vi "ATS9350_AsyncDMA.vi"() -> ()   [LabVIEW 2012]
doc: "ATS_AutoDMA.vi:\nExample of using the AutoDMA mode."
uses:
  ATS_ctl/ATS_DMA_Channel.ctl
  ATS_ctl/ATS_ReadSamples.ctl
  ATS_ctl/Device_Ctrl.ctl
  ATS_ctl/ATS_Async_Ctrl.ctl
  ATS_ctl/ATS_Check_Ctrl.ctl
  ATS_ctl/ClockSource.ctl
  ATS_ctl/ClockEdge.ctl
  ATS_ctl/Coupling.ctl
  ATS_ctl/Impedance.ctl
  ATS_ctl/TriggerOperation.ctl
  ATS_ctl/Bandwidth.ctl
  ATS_ctl/ExtTrigRange.ctl
  ATS_ctl/ATS_Async_Setting.ctl
  ATS_ctl/ATS_Async_Mode.ctl
panel:
  in  "Case Constant\n(See Context Help)":bool=TRUE
  in  "GetProcessedData":bool=TRUE
  in  "DataBuffer":bool
  out "Board":string
  in  "VersionC":bool caption="Version"
  out "Version":string=" "
  in  "Buffer Count":i32
  in  "StopCapture":bool
  in  "Tab Control":T1(tab)=enum."NPT"
  in  "Trad_ReadSamples":T2={"Offset"=0, "Length"=8192} caption="ReadSamples"
  in  "Trad_Records":u32=100 caption="Total Records"
  in  "Trad_RecPerBuf":u32=1 caption="RecPerBuf"
  out "NPT_BufferSize":u32=1024000 caption="BufferSize"
  in  "NPT_RecLength":u32=8192 caption="Record Length"
  in  "NPT_TotalRecords":u32=10000 caption="Total Records"
  in  "NPT_RecPerBuf":u32=125 caption="Records Per Buffer"
  in  "CT_Records":u32=100 caption="Total Records"
  in  "CT_BufferSize":u32=1024000 caption="Buffer Size"
  in  "TR_Records":u32=100 caption="Total Records"
  in  "Trig_BufferSize":u32=1024000 caption="Buffer Size"
  in  "SetupDMA":bool
  out "Error":string
  out "cFlags":u32 format="%x"
  out "SR (S/s)":dbl=10000000.0 format="%.2p"
  out "#Records":i32
  out "#Valid Buffer":i32
  out "ready":bool
  in  "SetBoard":bool
  in  "StartCapture":bool
  in  "Display":bool
  in  "Write TO file":bool
  out "#Loop":i32
  out "Time (ms)":u32
  out "Waveform Graph":u16[][](graph)
  out "Return Code":u32
  out "ReadSamples_Out":T2
  in  "Channel":T3
  in  "Device":i32
  in  "Stop":bool
  # "Total_Rec = 0 ==> Infini"
  # "Warning: Do not use ATS9462 in Traditional Mode"
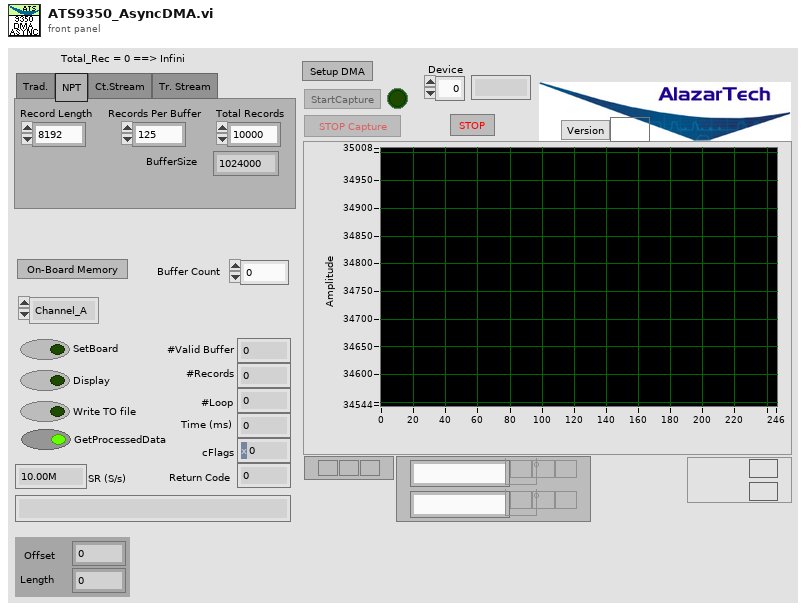
[diagram p1: front panel]
types:
  T1 = enum32{"Trad.", "NPT", "Ct.Stream", "Tr. Stream"}
  T2 = typedef "ATS_ReadSamples.ctl" = cluster{"Offset":i32, "Length":u32}
  T3 = typedef "ATS_DMA_Channel.ctl" = enum16{"Channel_A", "Channel_B", "A & B"}
  T4 = typedef "Device_Ctrl.ctl" = enum16{"Status", "About", "Arm", "ForceTrig", "Abort", "Initialize", "Init (NoPreset)", "Info", "Close", "Calibrate", "SetManually", "LED_ON", "LED_OFF"}
  T5 = typedef "ATS_Async_Ctrl.ctl" = enum16{"SetupDMA", "StartCapture", "Get", "Get_Stream", "Abort", "Stop"}
  T6 = typedef "ATS_Check_Ctrl.ctl" = enum16{"None", "NO_ATS9462", "ATS9462_Traditional", "Verify Board", "OnBoard Memory", "Board & Memory", "Master/Slave", "NO Master/Slave"}
  T7 = typedef "ATS_Async_Setting.ctl" = cluster{"UseHeader":u32, "Rec/Buffer":u32, "Total_Rec":u32, "DataBuffer":bool, "GetProcessedData":bool}
  T8 = typedef "ATS_Async_Mode.ctl" = enum16{"Continuous", "Triggered", "No-Pre-Trigger", "Traditional"}
  T9 = cluster{"Stop":bool, "Write TO file":bool, "SetBoard":bool, "StartDMA":bool, "StartCapture":bool, "Version":bool}
  T10 = cluster{"Stop":bool, "Write TO file":bool, "SetBoard":bool, "SetupDMA":bool, "StartCapture":bool, "VersionC":bool}
  T11 = cluster{"Stop":bool, "Write TO file":bool, "SetBoard":bool, bool, "StartCapture":bool, bool}
  T12 = typedef "ATS_Global.ctl" = cluster{"Record":T13, "Clock":T14, "Input A":T18, "Input B":T18, "Trigger":T23}
  T13 = typedef "Record.ctl" = cluster{"Count":u32, "Presize":u32, "Length":u32}
  T14 = typedef "Clock.ctl" = cluster{"ClckSource":T15, "ClckRate":T16, "ClckEdge":T17, "Decimation":u32}
  T15 = typedef "ClockSource.ctl" = enum16{"Internal", "External", "Medium Ext.", "Slow Ext.", "Ext. AC", "Ext. DC", "Ext. (PLL)"}
  T16 = typedef "ClockRate.ctl" = u32
  T17 = typedef "ClockEdge.ctl" = u16
  T18 = typedef "InputCtrl.ctl" = cluster{"Coupling":T19, "Range":T20, "Impedance":T21, "Bandwidth":T22}
  T19 = typedef "Coupling.ctl" = enum16{"AC", "DC"}
  T20 = typedef "Range.ctl" = u32
  T21 = typedef "Impedance.ctl" = enum16{"1M ohms", "50 ohms"}
  T22 = typedef "Bandwidth.ctl" = enum16{"Full Bandwidth", "Reduce Bandwidth"}
  T23 = typedef "Trigger.ctl" = cluster{"TrigOperation":T24, "Timeout (s)":dbl, "Trig. Delay":u32, "Engine X":T25, "Engine Y":T25, "ExtTrigControl":T26}
  T24 = typedef "TriggerOperation.ctl" = enum16{"Only X", "Only Y", "X or Y", "X and Y", "X xor Y", "X and not Y", "not X and Y"}
  T25 = typedef "TriggerEngine.ctl" = cluster{"Source":enum32{"Chan_A", "Chan_B", "External", "Disable"}, "Slope":enum32{"Positive", "Negative"}, "Level":u32}
  T26 = typedef "ExtTrigger.ctl" = cluster{"Coupling":T19, "Range":T27}
  T27 = typedef "ExtTrigRange.ctl" = enum16{"1 V", "5 V", "TTL"}
  T28 = cluster{"DeviceOut":i32, "Setup_Out":T12, "SR (S/s)":dbl, "Controls":cluster{"Stop":bool, "Write TO file":bool, "SetBoard":bool, "StartDMA":bool, "StartCapture":bool, "Version":bool}, "Flash":bool, "Record/Buf":u32, "BufCount_Out":i32}
  T29 = typedef "ATS_Async_Status.ctl" = cluster{"Start DMA":bool, "StartCapture":bool, "Valid":bool, "Completed":bool, "InProgress":bool, "Timeout":bool, "Overflow":bool, "Error":bool}
  T30 = typedef "Device_Info.ctl" = cluster{"Handle":u32, "Board":string, "CPLD":string, "MemorySize":u32, "SampleSize":u8, "ID":i32, "High_Memory":bool, "Chan/Board":u8}
  T31 = typedef "ATS_Global_Specs_Ctrl.ctl" = cluster{"ClckSource":cluster{"Internal":bool, "External":bool, "Medium Ext.":bool, "Slow Ext.":bool, "Ext. AC":bool, "Ext. DC":bool, "Ext. (PLL)":bool}, "ClckRate":cluster{"1 kS/s":bool, "2 kS/s":bool, "5 kS/s":bool, "10 kS/s":bool, "20 kS/s":bool, "50 kS/s":bool, "100 kS/s":bool, "200 kS/s":bool, "500 kS/s":bool, "1 MS/s":bool, "2 MS/s":bool, "5 MS/s":bool, "10 MS/s":bool, "20 MS/s":bool, "25 MS/s":bool, "50 MS/s":bool, "100 MS/s":bool, "125 MS/s":bool, "160 MS/s":bool, "180 MS/s":bool, "200 MS/s":bool, "250 MS/s":bool, "500 MS/s":bool, "1 GS/s":bool}, "ClckEdge":cluster{"Rising":bool, "Falling":bool}, "InputCoupling":cluster{"AC":bool, "DC":bool}, "InputRange":cluster{"20mV":bool, "40mV":bool, "50mV":bool, "80mV":bool, "100mV":bool, "200mV":bool, "400mV":bool, "500mV":bool, "800mV":bool, "1 V":bool, "2 V":bool, "4 V":bool, "5 V":bool, "8 V":bool, "10 V":bool, "16 V":bool, "20 V":bool, "40 V":bool, "HiFi":bool, "1.25 V":bool}, "Impedance":cluster{"1M ohms":bool, "50 ohms":bool, "300 ohms":bool}, "Bandwidth":cluster{"Full":bool, "Reduce":bool}, "RangeLim(50)":string, "AsyncDMA":cluster{"OnBoard":bool, "FPGA":bool}, "Memory":cluster{"VerifMem":bool, "HighMem":bool, "Combine":bool, "HighRecord":bool}, "ExtTrigCoupling":cluster{"AC":bool, "DC":bool}, "ExtTrigRange":cluster{"1 V":bool, "5 V":bool, "\nTTL":bool}, "AUX_IO_Trig":cluster{"Trig_Out":bool, "Trig_In":bool}, "AUX_IO_Slope":cluster{"Rising":bool, "Falling":bool}, "MaxPretrig":cluster{"MEM":u32, "FIFO":u32}, "AUX_I/O_Trig":cluster{"OUT_Trigger":bool, "OUT_PACER":bool, "OUT_BUSY":bool, "OUT_CLOCK":bool, "OUT_RESERVED":bool, "OUT_CAPTURE_ALMOST_DONE":bool, "OUT_AUXILIARY":bool, "OUT_SERIAL_DATA":bool, "IN_TRIGGER_ENABLE":bool, "IN_DIGITAL_TRIGGER":bool, "IN_GATE":bool, "IN_CAPTURE_ON_DEMAND":bool, "IN_RESET_TIMESTAMP":bool, "IN_SLOW_EXTERNAL_CLOCK":bool, "INPUT_AUXILIARY":bool, "INPUT_SERIAL_DATA":bool}, "ChannelsPerBoard":u8}
  T32 = enum32{"Chan_A", "Chan_B", "External", "Disable"}
  T33 = cluster{"Coupling":T19, "9350_Range":u32, "Impedance":T21, "Bandwidth":T22}
  T34 = cluster{"ClckSource":T15, "9350_ClckRate":u32, "ClckEdge":T17, "Decimation":u32}
  T35 = cluster{"Source":enum32{"Chan_A", "Chan_B", "External", "Disable"}, "Slope":enum32{"Positive", "Negative"}, "Level":u32}
  T36 = cluster{"Engine Relationship":T24, "Timeout (s)":dbl, "Trig. Delay":u32, cluster{"Source":enum32{"Chan_A", "Chan_B", "External", "Disable"}, "Slope":enum32{"Positive", "Negative"}, "Level":u32}, cluster{"Source":enum32{"Chan_A", "Chan_B", "External", "Disable"}, "Slope":enum32{"Positive", "Negative"}, "Level":u32}, cluster{"Coupling":T19, "Range":T27}}
  T37 = cluster{cluster{"Count":u32, "Offset":i32, "Length":u32}, cluster{"ClckSource":T15, "9350_ClckRate":u32, "ClckEdge":T17, "Decimation":u32}, cluster{"Coupling":T19, "9350_Range":u32, "Impedance":T21, "Bandwidth":T22}, cluster{"Coupling":T19, "9350_Range":u32, "Impedance":T21, "Bandwidth":T22}, cluster{"Engine Relationship":T24, "Timeout (s)":dbl, "Trig. Delay":u32, cluster{"Source":enum32{"Chan_A", "Chan_B", "External", "Disable"}, "Slope":enum32{"Positive", "Negative"}, "Level":u32}, cluster{"Source":enum32{"Chan_A", "Chan_B", "External", "Disable"}, "Slope":enum32{"Positive", "Negative"}, "Level":u32}, cluster{"Coupling":T19, "Range":T27}}}
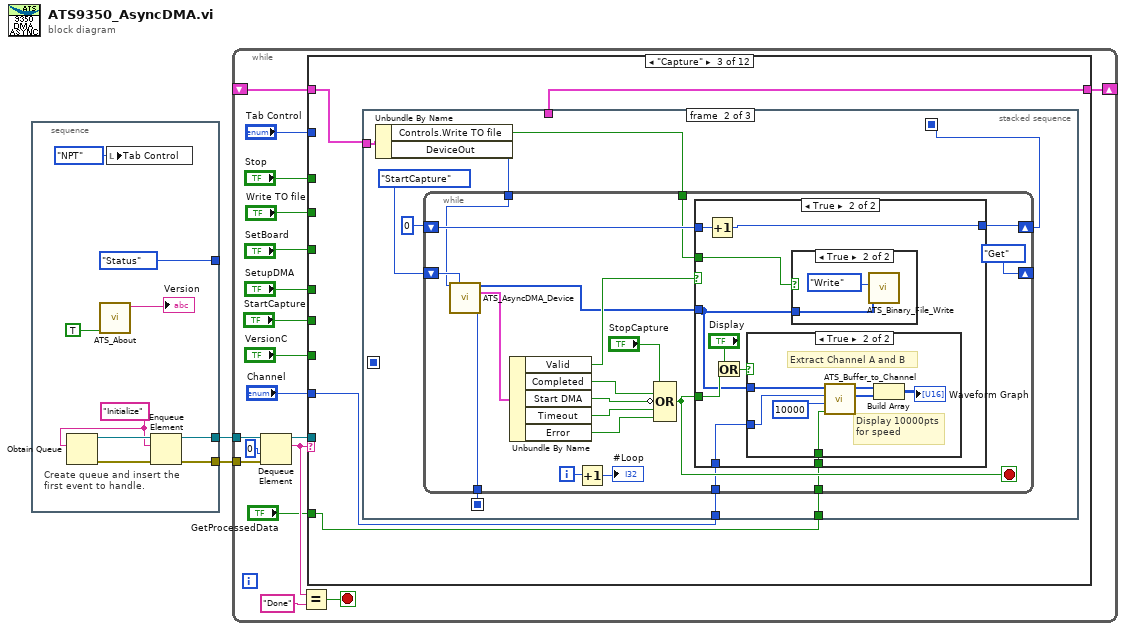
[diagram p0: block diagram]
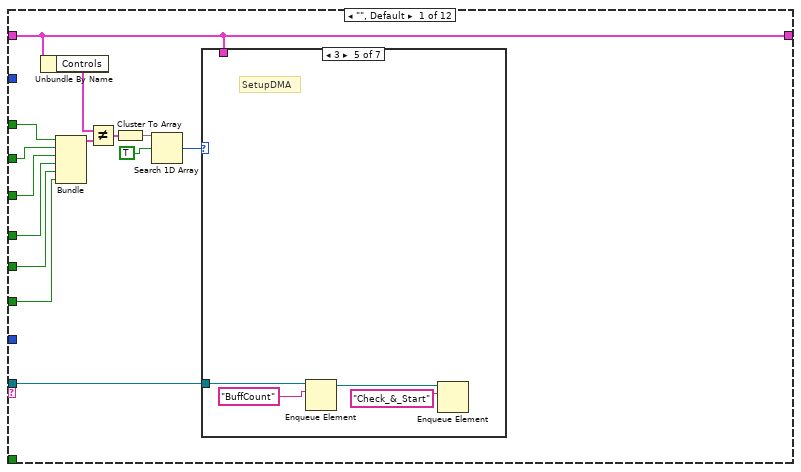
[diagram p2: hidden frame]
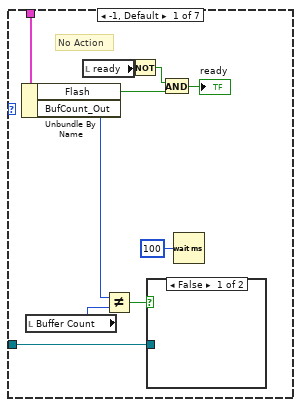
[diagram p3: hidden frame]
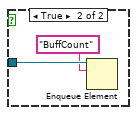
[diagram p4: hidden frame]
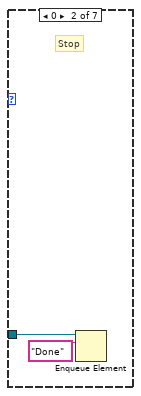
[diagram p5: hidden frame]
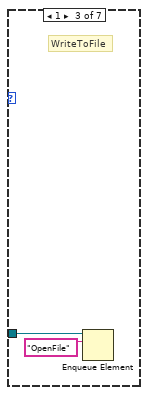
[diagram p6: hidden frame]
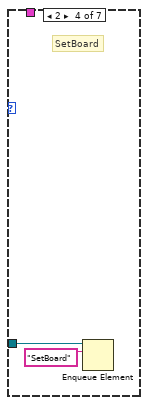
[diagram p7: hidden frame]
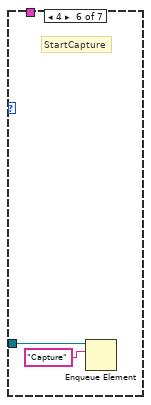
[diagram p8: hidden frame]
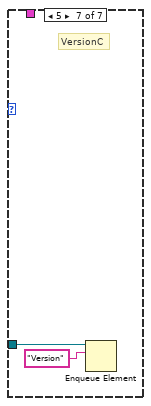
[diagram p9: hidden frame]
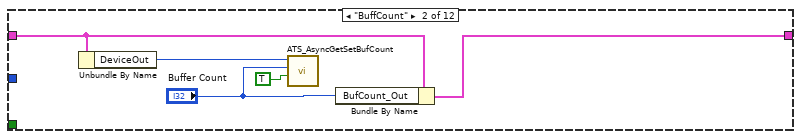
[diagram p10: hidden frame]
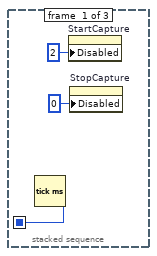
[diagram p11: hidden frame]
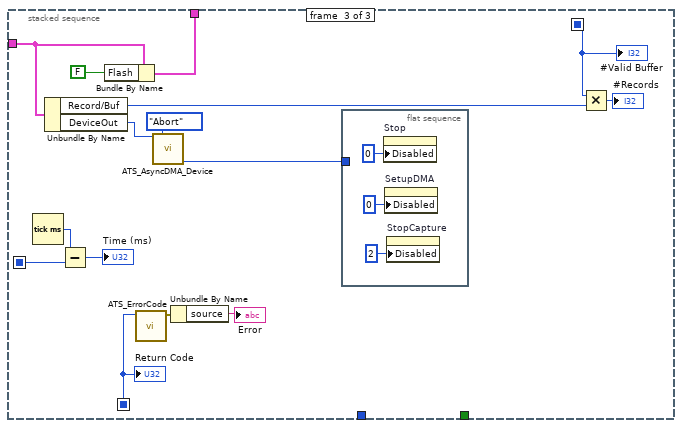
[diagram p15: hidden frame]
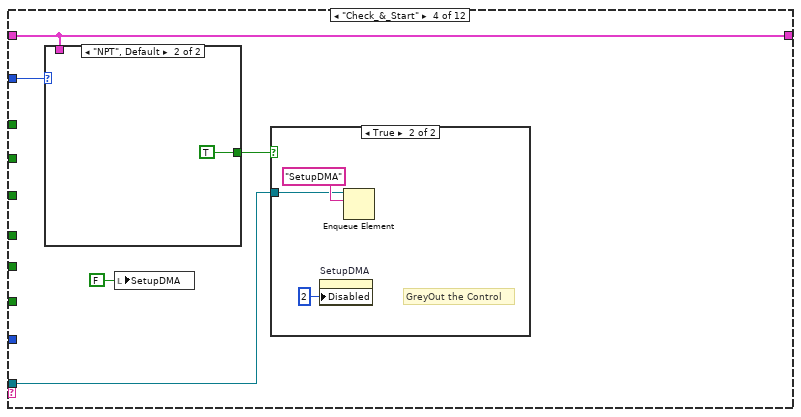
[diagram p16: hidden frame]
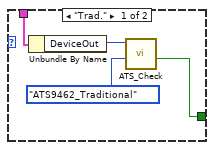
[diagram p18: hidden frame]
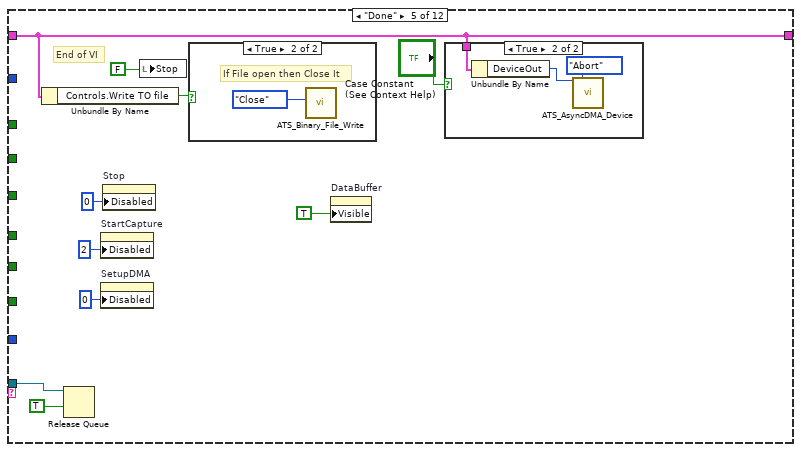
[diagram p19: hidden frame]
diagram:
  n1 = stacked-sequence {
    tunnel: [Device_Ctrl."Status" ("DevCtrl")] -> _
    tunnel: [w8] -> w2
    tunnel: [w7] -> w1
    frame #0 {
      w5 = "Initialize"
      # "Create queue and insert the\nfirst event to handle."
      n2 = Obtain Queue(element data type=w5) -> (queue out=w6:refnum<queue>, error out=w9:errorcluster)  [unwired: 4 in, 1 out]
      n3 = call "ATS_About.vi"("NO Display"=TRUE) -> ("Version#"=→"Version":string)  [unwired: 5 in, 1 out]
      n4 = local write "Tab Control"(T1."NPT" ("Tab Control")) -> ()
      n5 = Enqueue Element(queue=w6, element=w5, error in (no error)=w9) -> (queue out=w8:refnum<queue>, error out=w7:errorcluster)  [unwired: 1 in, 1 out]
    }
  }
  n6 = while {
    tunnel: w2 -> [w27]
    tunnel: w1 -> [w28]
    shift-right: [w22] -> _
    shift-left: _ -> [w21]
    stop <- w26 stop-if-true
    n7 = Dequeue Element(queue=w27, timeout in ms (-1)=0 ("ms timeout (-1)"), error in (no error)=w28) -> (queue out=w23:refnum<queue>, element=w24:string)  [unwired: 2 out]
    n8 = Equal?(x=w24, y="Done") -> (x = y?=w26:bool)
    n9 = case shown="\"Capture\"" w24 {
      tunnel: w23 -> [w35 _ _ w150 w170 w207 _ w254 w262 _ w344 _]
      tunnel: [w31 w73 w77 w152 w167 w204 w217 w257 w266 w292 w348 w350] -> w22
      tunnel: w21 -> [w31 w74 w78 w152 w167 _ w218 w253 w261 w293 w348 w350]
      tunnel: "Write TO file" -> [w43 _ _ _ _ _ w216 _ _ _ _ _]
      tunnel: "SetBoard" -> [w42 _ _ _ _ _ _ _ _ _ _ _]
      tunnel: "SetupDMA" -> [w34 _ _ _ _ _ _ _ _ _ _ _]
      tunnel: "Stop" -> [w33 _ _ _ _ _ _ _ _ _ _ _]
      tunnel: "StartCapture" -> [w32 _ _ _ _ _ _ _ _ _ _ _]
      tunnel: "Channel" -> [_ _ w76 _ _ _ _ _ _ w289 _ _]
      tunnel: "Tab Control" -> [_ _ _ w151 _ _ _ _ _ w271 _ _]
      tunnel: "VersionC" -> [w30 _ _ _ _ _ _ _ _ _ _ _]
      tunnel: "GetProcessedData" -> [_ _ w75 _ _ _ _ _ _ w270 _ _]
      frame "", Default {
        n10 = Unbundle By Name(w31) -> ("Controls"=w40:T9)
        n11 = Bundle("Stop"=w33, "Write TO file"=w43, "SetBoard"=w42, "SetupDMA"=w34, "StartCapture"=w32, "VersionC"=w30) -> (w41:T10)  [unwired: 1 in]
        n12 = Not Equal?(x=w40, y=w41) -> (x != y?=w39:T11)
        n13 = Cluster To Array(cluster=w39) -> (array=w37:bool[])
        n14 = Search 1D Array(1D array=w37, element=TRUE) -> (index of element=w36:i32)  [unwired: 1 in]
        n15 = case shown="3" w36 {
          tunnel: w35 -> [w44 w57 w58 w60 w65 w66 w68]
          tunnel: w31 -> [w52 _ _ _ _ _ _]
          frame -1, Default {
            # "No Action"
            n16 = Unbundle By Name(w52) -> ("Flash"=w49:bool, "BufCount_Out"=w47:i32)
            n17 = local read "Buffer Count"() -> (w46:i32)
            n18 = local read "ready"() -> (w51:bool)
            n19 = Not Equal?(x=w47, y=w46) -> (x != y?=w45:bool)
            n20 = Not(x=w51) -> (.not. x?=w48:bool)
            n21 = case shown="False" w45 {
              tunnel: w44 -> [_ w55]
              frame False {
              }
              frame True {
                n22 = Enqueue Element(queue=w55, element="BuffCount") -> ()  [unwired: 2 in, 3 out]
              }
            }
            n23 = And(x=w48, y=w49) -> (x .and. y?=→"ready":bool)
            n24 = Wait (ms)(milliseconds to wait=u32 100) -> ()  [unwired: 1 out]
          }
          frame 0 {
            # "Stop"
            n25 = Enqueue Element(queue=w57, element="Done") -> ()  [unwired: 2 in, 3 out]
          }
          frame 1 {
            # "WriteToFile"
            n26 = Enqueue Element(queue=w58, element="OpenFile") -> ()  [unwired: 2 in, 3 out]
          }
          frame 2 {
            # "SetBoard"
            n27 = Enqueue Element(queue=w60, element="SetBoard") -> ()  [unwired: 2 in, 3 out]
          }
          frame 3 {
            # "SetupDMA"
            n28 = Enqueue Element(queue=w65, element="BuffCount") -> (queue out=w62:refnum<queue>)  [unwired: 2 in, 2 out]
            n29 = Enqueue Element(queue=w62, element="Check_&_Start") -> ()  [unwired: 2 in, 3 out]
          }
          frame 4 {
            # "StartCapture"
            n30 = Enqueue Element(queue=w66, element="Capture") -> ()  [unwired: 2 in, 3 out]
          }
          frame 5 {
            # "VersionC"
            n31 = Enqueue Element(queue=w68, element="Version") -> ()  [unwired: 2 in, 3 out]
          }
        }
      }
      frame "BuffCount" {
        n32 = Unbundle By Name(w74) -> ("DeviceOut"=w72:i32)
        n33 = call "ATS_AsyncGetSetBufCount.vi"("Get / Set&Get"=TRUE, "BuffCount"="Buffer Count", "DeviceIn"=w72) -> ()  [unwired: 6 in, 3 out]
        n34 = Bundle By Name(cluster=w74, "BufCount_Out"="Buffer Count") -> (w73:T28)
      }
      frame "Capture" {
        n35 = stacked-sequence {
          seq-local: [w81 _ _] -> [_ _ w142]
          seq-local: [_ w85 _] -> [_ _ w132]
          seq-local: [_ w83 _] -> [_ _ w131]
          tunnel: w78 -> [_ w88 w137]
          tunnel: [_ _ w140] -> w77
          tunnel: w76 -> [_ w84 _]
          tunnel: w75 -> [_ w82 _]
          frame #0 {
            n36 = Tick Count (ms)() -> (millisecond timer value=w81:u32)
            n37 = property on="StartCapture" class="Bool"("Disabled"=u8 2) -> ()  [unwired: 2 in, 2 out]
            n38 = property on="StopCapture" class="Bool"("Disabled"=u8 0) -> ()  [unwired: 2 in, 2 out]
          }
          frame #1 {
            n39 = Unbundle By Name(w88) -> ("Controls.Write TO file"=w86:bool, "DeviceOut"=w87:i32)
            n40 = while {
              shift-right: [w101] -> w83
              shift-left: 0 -> [w105]
              shift-right: [ATS_Async_Ctrl."Get" ("ATS_DMA_Ctrl")] -> _
              shift-left: ATS_Async_Ctrl."StartCapture" ("ATS_DMA_Ctrl") -> [w99]
              tunnel: [w97] -> w85
              tunnel: w87 -> [w96]
              tunnel: w86 -> [w95]
              tunnel: w84 -> [w94]
              tunnel: w82 -> [w91]
              i -> [w106]
              stop <- w103 stop-if-true
              n41 = call "ATS_AsyncDMA_Device.vi"("DeviceIn"=w96, "ATS_Async_Ctrl"=w99) -> ("Buffer"=w107:u16[], "Async_Status"=w92:T29, "Return Code"=w97:u32)  [unwired: 9 in, 2 out]
              n42 = Unbundle By Name(w92) -> ("Valid"=w110:bool, "Completed"=w104:bool, "Start DMA"=w109:bool, "Timeout"=w108:bool, "Error"=w98:bool)
              n43 = Increment(x=w106) -> (x+1=→"#Loop":i32)
              n44 = Compound Arithmetic op=OR("StopCapture", w104, invert w109, w108, w98) -> (w103:bool)
              n45 = case shown="True" w110 {
                tunnel: w107 -> [_ w115]
                tunnel: w95 -> [_ w120]
                tunnel: w105 -> [w111 w118]
                tunnel: [w111 w114] -> w101
                tunnel: w103 -> [_ w116]
                tunnel: w94 -> [_ w113]
                tunnel: w91 -> [_ w112]
                frame False {
                }
                frame True {
                  n46 = Increment(x=w118) -> (x+1=w114:i32)
                  n47 = Or(x="Display", y=w116) -> (x .or. y?=w117:bool)
                  n48 = case shown="True" w117 {
                    tunnel: w115 -> [_ w123]
                    tunnel: w113 -> [_ w122]
                    tunnel: w112 -> [_ w121]
                    frame False {
                    }
                    frame True {
                      # "Extract Channel A and B"
                      # "Display 10000pts\nfor speed"
                      n49 = call "ATS_Buffer_to_Channel.vi"("GetProcessedData"=w121, "MaxLength (-1)"=10000 ("length"), "Channel"=w122, "Buffer [AB]"=w123) -> ("[B]"=w126:u16[], "[A]"=w127:u16[])  [unwired: 6 in]
                      n50 = Build Array(w127, w126) -> (→"Waveform Graph":u16[][])
                    }
                  }
                  n51 = case shown="True" w120 {
                    tunnel: w115 -> [_ w128]
                    frame False {
                    }
                    frame True {
                      n52 = call "ATS_Binary_File_Write.vi"("Data_In"=w128, "Write_Ctrl"=enum16{"Open", "Write", "Close"}."Write") -> ()  [unwired: 8 in, 2 out]
                    }
                  }
                }
              }
            }
          }
          frame #2 {
            n53 = Tick Count (ms)() -> (millisecond timer value=w144:u32)
            n54 = Unbundle By Name(w137) -> ("Record/Buf"=w135:u32, "DeviceOut"=w134:i32)
            n55 = Subtract(x=w144, y=w142) -> (x-y=→"Time (ms)":u32)
            n56 = Bundle By Name(cluster=w137, "Flash"=FALSE) -> (w140:T28)
            n57 = call "ATS_ErrorCode.vi"("ErrorCode"=w132) -> ("error out"=w133:errorcluster)  [unwired: 6 in]
            n58 = call "ATS_AsyncDMA_Device.vi"("DeviceIn"=w134, "ATS_Async_Ctrl"=ATS_Async_Ctrl."Abort" ("ATS_DMA_Ctrl")) -> ("Return Code"=w130:u32)  [unwired: 9 in, 4 out]
            n59 = Unbundle By Name(w133) -> ("source"=→"Error":string)
            n60 = flat-sequence {
              tunnel: w130 -> [_]
              frame #0 {
                n61 = property on="Stop" class="Bool (strict)"("Disabled"=u8 0) -> ()  [unwired: 2 in, 2 out]
                n62 = property on="SetupDMA" class="Bool (strict)"("Disabled"=u8 0) -> ()  [unwired: 2 in, 2 out]
                n63 = property on="StopCapture" class="Bool"("Disabled"=u8 2) -> ()  [unwired: 2 in, 2 out]
              }
            }
            n64 = Multiply(x=w131, y=w135) -> (x*y=→"#Records":u32)
            "Return Code" <- w132
            "#Valid Buffer" <- w131
          }
        }
      }
      frame "Check_&_Start" {
        n65 = case shown="\"NPT\", Default" w151 {
          tunnel: w152 -> [w159 _]
          tunnel: [w157 TRUE ("OK")] -> w149
          frame "Trad." {
            n66 = Unbundle By Name(w159) -> ("DeviceOut"=w158:i32)
            n67 = call "ATS_Check.vi"("ATS_Check"=ATS_Check_Ctrl."ATS9462_Traditional", "Device"=w158) -> ("OK"=w157:bool)  [unwired: 8 in, 1 out]
          }
          frame "NPT", Default {
          }
        }
        n68 = local write "SetupDMA"(FALSE ("StartDMA")) -> ()
        n69 = case shown="True" w149 {
          tunnel: w150 -> [_ w154]
          frame False {
          }
          frame True {
            # "GreyOut the Control"
            n70 = property on="SetupDMA" class="Bool (strict)"("Disabled"=u8 2) -> ()  [unwired: 2 in, 2 out]
            n71 = Enqueue Element(queue=w154, element="SetupDMA") -> ()  [unwired: 2 in, 3 out]
          }
        }
      }
      frame "Done" {
        # "End of VI"
        n72 = Unbundle By Name(w167) -> ("Controls.Write TO file"=w168:bool)
        n73 = Release Queue(queue=w170, force destroy? (F)=TRUE) -> ()  [unwired: 1 in, 3 out]
        n74 = property on="StartCapture" class="Bool"("Disabled"=u8 2) -> ()  [unwired: 2 in, 2 out]
        n75 = property on="SetupDMA" class="Bool (strict)"("Disabled"=u8 0) -> ()  [unwired: 2 in, 2 out]
        n76 = property on="Stop" class="Bool (strict)"("Disabled"=u8 0) -> ()  [unwired: 2 in, 2 out]
        n77 = local write "Stop"(FALSE ("Stop")) -> ()
        n78 = case shown="True" w168 {
          frame False {
          }
          frame True {
            # "If File open then Close It"
            n79 = call "ATS_Binary_File_Write.vi"("Write_Ctrl"=enum16{"Open", "Write", "Close"}."Close" ("f")) -> ()  [unwired: 9 in, 2 out]
          }
        }
        n80 = property on="DataBuffer" class="Bool (strict)"("Visible"=TRUE) -> ()  [unwired: 2 in, 2 out]
        n81 = case shown="True" "Case Constant\n(See Context Help)" {
          tunnel: w167 -> [_ w172]
          frame False {
          }
          frame True {
            n82 = Unbundle By Name(w172) -> ("DeviceOut"=w171:i32)
            n83 = call "ATS_AsyncDMA_Device.vi"("DeviceIn"=w171, "ATS_Async_Ctrl"=ATS_Async_Ctrl."Abort" ("ATS_DMA_Ctrl")) -> ()  [unwired: 9 in, 5 out]
          }
        }
      }
      frame "Initialize" {
        w190 = u32 0  # Record/Buf
        w203 = T9 {"Stop"=FALSE, "Write TO file"=FALSE, "SetBoard"=FALSE, "StartDMA"=FALSE, "StartCapture"=FALSE, "Version"=FALSE}  # Controls
        w192 = FALSE  # Flash
        # "Reset all Boards"
        n84 = Enqueue Element(queue=w207, element="PreSet" ("queue element")) -> ()  [unwired: 2 in, 3 out]
        n85 = call "ATS_Device.vi"("BoardToVerify"="ATS9350", "ATS_Check"=ATS_Check_Ctrl."Verify Board", "DevCtrl"=Device_Ctrl."Initialize", "DeviceIn"="Device") -> ("DeviceOut"=w209:i32, "DevInfo"=w186:T30)  [unwired: 1 in, 5 out]
        n86 = local write "#Valid Buffer"(0 ("#Valid Buffer")) -> ()
        n87 = local write "#Records"(0 ("#Records")) -> ()
        n88 = Unbundle By Name(w186) -> ("Board"=→"Board":string)
        n89 = property on="StartCapture" class="Bool"("Disabled"=u8 2) -> ()  [unwired: 2 in, 2 out]
        n90 = property on="StopCapture" class="Bool"("Disabled"=u8 2) -> ()  [unwired: 2 in, 2 out]
        n91 = property on="SetupDMA" class="Bool (strict)"("Disabled"=u8 0) -> ()  [unwired: 2 in, 2 out]
        n92 = local write "Time (ms)"(u32 0 ("TimeLoop (ms)")) -> ()
        n93 = property on="Stop" class="Bool (strict)"("Disabled"=u8 0) -> ()  [unwired: 2 in, 2 out]
        n94 = call "ATS_Device.vi"("DevCtrl"=Device_Ctrl."Abort", "DeviceIn"=w209) -> ("DeviceOut"=w181:i32)  [unwired: 3 in, 6 out]
        n95 = call "ATS_Specs_Selection.vi"("Device"=w181) -> ("Specifications"=w180:T31)  [unwired: 4 in, 6 out]
        n96 = call "ATS_MS_Set_Device.vi"("Update_Only"=TRUE ("Set_Manually (F)"), "DeviceIn"=w181) -> ("Setup_Out"=w194:T12, "DeviceOut"=w188:i32)  [unwired: 4 in, 4 out]
        n97 = Unbundle By Name(w180) -> ("AsyncDMA.OnBoard"=w179:bool, "AsyncDMA.FPGA"=w175:bool)
        n98 = call "ATS_AsyncGetSetBufCount.vi"("DeviceIn"=w188) -> ("BufCount_Out"=w187:i32)  [unwired: 8 in, 2 out]
        n99 = local read "SR (S/s)"() -> (w205:dbl)
        n100 = And(x=w179, y=w175) -> (x .and. y?=w178:bool)
        n101 = Unbundle By Name(w203) -> ("Stop"=w196:bool, "Write TO file"=w202:bool, "SetBoard"=w201:bool, "StartDMA"=w197:bool)
        n102 = case shown="False" w178 {
          selector: w178 -> [w213 w215]
          tunnel: [w213 w215] -> w177
          tunnel: [w212 w214] -> w176
          tunnel: w175 -> [w212 w214]
          frame False {
          }
          frame True {
          }
        }
        n103 = local write "Buffer Count"(w187) -> ()
        n104 = Bundle("DeviceOut"=w181, "Setup_Out"=w194, "SR (S/s)"=w205, "Controls"=w203, "Flash"=w192, "Record/Buf"=w190, "BufCount_Out"=w187) -> (w204:T28)  [unwired: 1 in]
        n105 = local write "SetupDMA"(w197) -> ()
        n106 = local write "Write TO file"(w202) -> ()
        n107 = local write "SetBoard"(w201) -> ()
        n108 = local write "Stop"(w196) -> ()
        n109 = property on="DataBuffer" class="Bool (strict)"("Visible"=w177, "Value"=w176) -> ()  [unwired: 2 in, 2 out]
      }
      frame "OpenFile" {
        n110 = Select(t=enum16{"Open", "Write", "Close"}."Open" ("Write_Ctrl"), s=w216, f=enum16{"Open", "Write", "Close"}."Close") -> (s? t:f=w220:enum16{"Open", "Write", "Close"})
        n111 = Bundle By Name(cluster=w218, "Controls.Write TO file"=w216) -> (w217:T28)
        n112 = call "ATS_Binary_File_Write.vi"("Write_Ctrl"=w220) -> ()  [unwired: 9 in, 2 out]
      }
      frame "PreSet" {
        w243 = enum32{"Positive", "Negative"}."Positive"  # Slope
        w242 = enum32{"Positive", "Negative"}."Positive"  # Slope
        w241 = T32."Disable"  # Source
        w239 = T32."Chan_A"  # Source
        w223 = u32 4 items=["40mV", "100mV", "200mV", "400mV", "1 V", "2 V", "4 V"]  # 9350_Range
        w222 = u32 17 items=["1 kS/s", "2 kS/s", "5 kS/s", "10 kS/s", "20 kS/s", "50 kS/s", "100 kS/s", "200 kS/s", "500 kS/s", "1 MS/s", "2 MS/s", "5 MS/s", "10 MS/s", "20 MS/s", "50 MS/s", "100 MS/s", "250 MS/s", "500 MS/s"]  # 9350_ClckRate
        w248 = ExtTrigRange."1 V"  # Range
        w247 = Coupling."AC"  # Coupling
        w246 = Bandwidth."Full Bandwidth"  # Bandwidth
        w245 = u32 0  # Decimation
        w244 = u32 1  # Count
        w227 = u32 0  # Trig. Delay
        w228 = TriggerOperation."Only X"  # Engine Relationship
        w226 = 0.0  # Timeout (s)
        w240 = u32 150  # Level
        w234 = Impedance."50 ohms"  # Impedance
        w232 = Coupling."DC"  # Coupling
        w231 = T17 0 items=["Rising", "Falling"]  # ClckEdge
        w230 = ClockSource."Internal"  # ClckSource
        n113 = Unbundle By Name(w253) -> ("DeviceOut"=w256:i32)
        n114 = Enqueue Element(queue=w254, element="Update" ("queue element")) -> ()  [unwired: 2 in, 3 out]
        n115 = local read "Trad_ReadSamples"() -> (w224:T2)
        n116 = Bundle("Coupling"=w232, "9350_Range"=w223, "Impedance"=w234, "Bandwidth"=w246) -> (w233:T33)  [unwired: 1 in]
        n117 = Bundle("ClckSource"=w230, "9350_ClckRate"=w222, "ClckEdge"=w231, "Decimation"=w245) -> (w235:T34)  [unwired: 1 in]
        n118 = Unbundle By Name(w224) -> ("Offset"=w251:i32, "Length"=w250:u32)
        n119 = Bundle "EngineX"("Source"=w239, "Slope"=w243, "Level"=w240) -> (w237:T35)  [unwired: 1 in]
        n120 = Bundle "EngineY"("Source"=w241, "Slope"=w242, "Level"=w240) -> (w238:T35)  [unwired: 1 in]
        n121 = Bundle("Count"=w244, "Offset"=w251, "Length"=w250) -> (w229:cluster{"Count":u32, "Offset":i32, "Length":u32})  [unwired: 1 in]
        n122 = Bundle "Ext Trig"("Coupling"=w247, "Range"=w248) -> (w249:cluster{"Coupling":T19, "Range":T27})  [unwired: 1 in]
        n123 = Bundle("Engine Relationship"=w228, "Timeout (s)"=w226, "Trig. Delay"=w227, w237, w238, w249) -> (w236:T36)  [unwired: 1 in]
        n124 = Bundle(w229, w235, w233, w233, w236) -> (w225:T37)  [unwired: 1 in]
        n125 = call "ATS_MS_Set_Device.vi"("Set_Manually (F)"=FALSE, "Setup_In"=w225, "DeviceIn"=w256) -> ("Clock_Value (s)"=w252:dbl, "Setup_Out"=w258:T12)  [unwired: 3 in, 4 out]
        n126 = Bundle By Name(cluster=w253, "Setup_Out"=w258, "SR (S/s)"=w252) -> (w257:T28)
      }
      frame "SetBoard" {
        n127 = Unbundle By Name(w261) -> ("DeviceOut"=w264:i32)
        n128 = Enqueue Element(queue=w262, element="Update" ("queue element")) -> ()  [unwired: 2 in, 3 out]
        n129 = local write "SetBoard"(FALSE ("SetBoard")) -> ()
        n130 = call "ATS_MS_Set_Device.vi"("Set_Manually (F)"=TRUE, "DeviceIn"=w264) -> ("Clock_Value (s)"=w265:dbl, "Setup_Out"=w267:T12)  [unwired: 4 in, 4 out]
        n131 = Bundle By Name(cluster=w261, "Setup_Out"=w267, "SR (S/s)"=w265) -> (w266:T28)
      }
      frame "SetupDMA" {
        n132 = case shown="\"NPT\", Default" w271 {
          tunnel: [w302 "Trad_RecPerBuf" u32 1 u32 1] -> w280
          tunnel: ["NPT_TotalRecords" "Trad_Records" "CT_Records" "TR_Records"] -> w281
          tunnel: [ATS_Async_Mode."No-Pre-Trigger" ("Async_Mode") ATS_Async_Mode."Traditional" ("Async_Mode") ATS_Async_Mode."Continuous" ("Async_Mode") ATS_Async_Mode."Triggered" ("Async_Mode")] -> w284
          tunnel: [u32 0 u32 0 u32 0 u32 0] -> w282
          tunnel: [0 ("Offset") w316 0 ("Offset") 0 ("Offset")] -> w287
          tunnel: ["NPT_RecLength" w315 "CT_BufferSize" "Trig_BufferSize"] -> w286
          tunnel: [TRUE ("Start Now / Wait") TRUE ("Start Now / Wait") TRUE ("Start Now / Wait") TRUE ("Start Now / Wait")] -> w269
          frame "NPT", Default {
            n133 = case shown="1, Default" "NPT_TotalRecords" {
              tunnel: "NPT_RecPerBuf" -> [w308 w311]
              tunnel: "NPT_TotalRecords" -> [_ w310]
              tunnel: [w308 w309] -> w302
              frame 0 {
              }
              frame 1, Default {
                n134 = Max & Min(x=w311, y=w310) -> (min(x,y)=w309:u32)  [unwired: 1 out]
                n135 = local write "NPT_RecPerBuf"(w309) -> ()
              }
            }
            n136 = Multiply(x=w302, y="NPT_RecLength") -> (x*y=→"NPT_BufferSize":u32)
          }
          frame "Trad." {
            n137 = Unbundle By Name("Trad_ReadSamples") -> ("Offset"=w316:i32, "Length"=w315:u32)
          }
          frame "Ct.Stream" {
          }
          frame "Tr. Stream" {
          }
        }
        n138 = local write "SetupDMA"(FALSE ("StartDMA")) -> ()
        n139 = Unbundle By Name(w293) -> ("DeviceOut"=w274:i32)
        n140 = Bundle By Name(cluster=T7 {"UseHeader"=0, "Rec/Buffer"=0, "Total_Rec"=0, "DataBuffer"=FALSE, "GetProcessedData"=FALSE} ("Async_Setting"), "UseHeader"=w282, "Rec/Buffer"=w280, "Total_Rec"=w281, "DataBuffer"="DataBuffer", "GetProcessedData"=w270) -> (w279:T7)
        n141 = Bundle By Name(cluster=T2 {"Offset"=0, "Length"=8192} ("Trad_ReadSamples"), "Offset"=w287, "Length"=w286) -> (w285:T2)
        n142 = call "ATS_AsyncDMA_Device.vi"("DeviceIn"=w274, "ATS_Async_Ctrl"=ATS_Async_Ctrl."SetupDMA" ("ATS_DMA_Ctrl"), "Async_Mode"=w284, "Async_Setting"=w279, "Channel"=w289, "ReadSamples"=w285, "Start Now / Wait"=w269) -> ("Async_Status"=w296:T29, "ReadSamples_Out"=w272:T2, "cFlags_Out"=→"cFlags":u32, "Return Code"=w276:u32)  [unwired: 4 in, 1 out]
        "ReadSamples_Out" <- w272
        n143 = case shown="\"Trad.\"" w271 {
          tunnel: w272 -> [w298 _]
          frame "Trad." {
            n144 = local write "Trad_ReadSamples"(w298) -> ()
          }
          frame "NPT", Default {
          }
        }
        n145 = call "ATS_ErrorCode.vi"("ErrorCode"=w276) -> ("error out"=w277:errorcluster)  [unwired: 6 in]
        n146 = local write "Return Code"(w276) -> ()
        n147 = Unbundle By Name(w277) -> ("source"=w278:string)
        n148 = Unbundle By Name(w296) -> ("Error"=w291:bool)
        n149 = local write "Error"(w278) -> ()
        n150 = Not(x=w291) -> (.not. x?=w290:bool)
        n151 = case shown="False" w291 {
          tunnel: [u8 2 ("Disabled") u8 0 ("Disabled")] -> w275
          tunnel: w274 -> [w334 _]
          frame False {
            n152 = call "ATS_AsyncGetSetBufCount.vi"("DeviceIn"=w334) -> ("BufCount_Out"=w335:i32)  [unwired: 8 in, 2 out]
            n153 = local write "#Valid Buffer"(0 ("#Valid Buffer")) -> ()
            n154 = local write "#Records"(0 ("#Records")) -> ()
            n155 = local write "#Loop"(0 ("#Loop")) -> ()
            n156 = property on="StartCapture" class="Bool"("Disabled"=u8 0) -> ()  [unwired: 2 in, 2 out]
            n157 = property on="Stop" class="Bool (strict)"("Disabled"=u8 0) -> ()  [unwired: 2 in, 2 out]
            n158 = local write "Time (ms)"(u32 0 ("TimeLoop (ms)")) -> ()
            n159 = local write "Buffer Count"(w335) -> ()
          }
          frame True {
          }
        }
        n160 = Bundle By Name(cluster=w293, "Flash"=w290, "Record/Buf"=w280) -> (w292:T28)
        n161 = property on="SetupDMA" class="Bool (strict)"("Disabled"=w275) -> ()  [unwired: 2 in, 2 out]
      }
      frame "Update" {
        n162 = Unbundle By Name(w348) -> ("SR (S/s)"=w347:dbl)
        n163 = Enqueue Element(queue=w344, element="BuffCount") -> ()  [unwired: 2 in, 3 out]
        n164 = Reciprocal(x=w347) -> (1/x=→"SR (S/s)":dbl)
      }
      frame "Version" {
        n165 = Unbundle By Name(w350) -> ("DeviceOut"=w349:i32)
        n166 = call "ATS_Device.vi"("DevCtrl"=Device_Ctrl."About", "DeviceIn"=w349) -> ()  [unwired: 3 in, 7 out]
      }
    }
  }
